vi "Data Access.vi"(8 "error in (no error)":errorcluster, 10 "Data Access Handler":refnum<class "Data Access Handler.lvclass">, 11 "DMM Config Msg in":refnum<class "DMM Config Msg.lvclass">) -> (0 "error out":errorcluster, 3 "DMM Config Msg out":refnum<class "DMM Config Msg.lvclass">)   [LabVIEW 2020, in "DMM Msg.lvlib" / "DMM Config Msg.lvclass"]
doc: "Expose class private data to the front panel while letting the Data Access Handler class act on the data."
uses:
  DMM Config Msg.lvclass
  C:/Current projects/WS/PPL/HDH.Actor Framework.Core.Msg.lvlibp/Flex Msg/Flex Msg.lvclass
  PPL/HDH.Actor Framework.Core.Msg.lvlibp/Flex Msg/Data Access Handlers/Data Access Handler/Data Access Handler.lvclass
  PPL/HDH.Driver.DMM.lvlibp/Controls/Ctl_Function.ctl
  PPL/HDH.Driver.DMM.lvlibp/Controls/Ctl_DigitResolution.ctl
  PPL/HDH.Actor Framework.Core.Publisher.lvlibp/Messages/Response Msg/Response Core/Controls/Ctl_SendFunction.ctl
  DMM Config Msg.lvclass/DMM Config Msg.ctl
  PPL/HDH.Actor Framework.Core.Instrument Handler.lvlibp/Messages/Instrument Msg/Instrument Msg.lvclass
  C:/Current projects/WS/PPL/HDH.Actor Framework.Core.Instrument Handler.lvlibp/Messages/Instrument Msg/Instrument Msg.lvclass
  PPL/HDH.Driver.DMM.lvlibp
  PPL/HDH.Actor Framework.Core.Publisher.lvlibp
panel:
  in  "Message Priority":enum16{"Low", "Normal", "High"}(ring)=enum."Normal"
  in  "Timeout if Waiting":i32=-1
  in  "Send Function":T1=enum."Await Reply"
  in  "Digit Resolution":T2=enum."5½"
  in  "Range":dbl
  in  "Function":T3
  in  "Cancel":bool
  in  "OK":bool
  # "Send details"
  # "Configuration details"
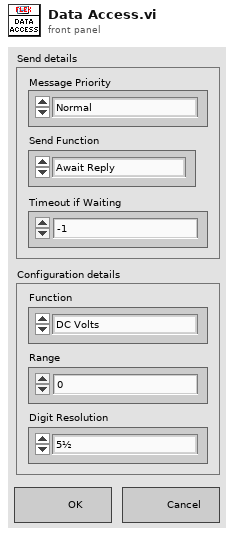
[diagram p1: front panel]
types:
  T1 = typedef "HDH.Actor Framework.Core.Publisher.lvlibp/Ctl_SendFunction.ctl" = enum16{"Send and Forget", "Request Reply", "Await Reply"}
  T2 = typedef "HDH.Driver.DMM.lvlibp/Ctl_DigitResolution.ctl" = enum8{"3½", "4½", "5½", "6½", "7½"}
  T3 = typedef "HDH.Driver.DMM.lvlibp/Ctl_Function.ctl" = enum8{"DC Volts", "AC Volts", "DC Current", "AC Current", "2-wire Resistance", "4-wire Resistance", "Diode", "Frequency", "Period", "AC Volts DC Coupled", "Capacitance", "Inductance", "Temperature"}
  T4 = typedef "HDH.Actor Framework.Core.Actor.lvlibp/Message Enqueuer.lvclass/Message Priority.ctl" = enum16{"Low", "Normal", "High"}
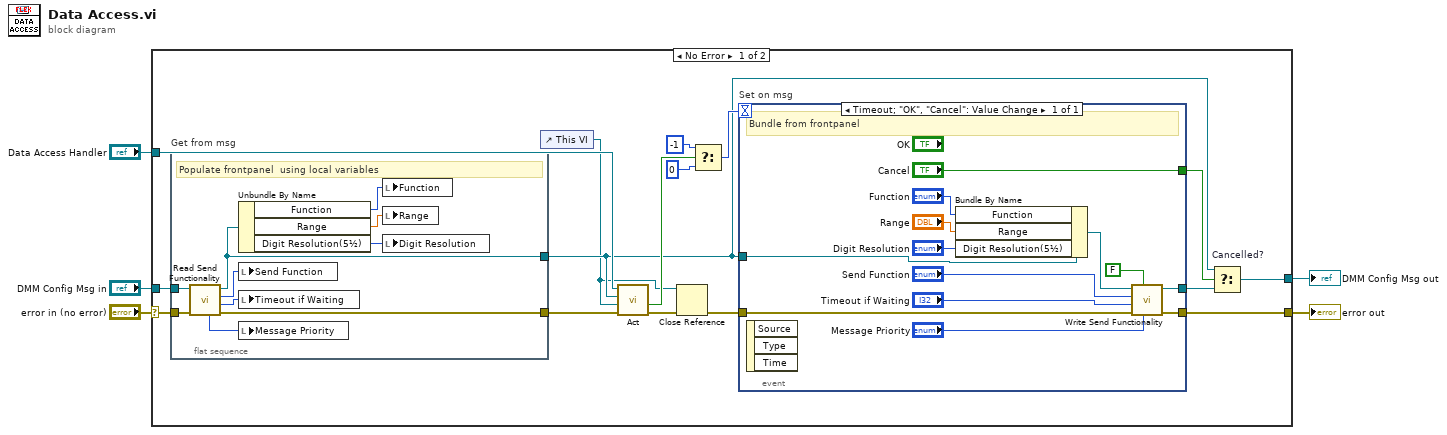
[diagram p0: block diagram]
diagram:
  n1 = case shown="No Error" "error in (no error)" {
    selector: "error in (no error)" -> [w21 w46]
    tunnel: [w14 w46] -> w4
    tunnel: [w9 w45] -> w2
    tunnel: "DMM Config Msg in" -> [w12 w45]
    tunnel: "Data Access Handler" -> [w20 _]
    frame No Error {
      n2 = flat-sequence "Get from msg" {
        tunnel: w21 -> [w43]
        tunnel: [w41] -> w7
        tunnel: w12 -> [w44]
        tunnel: [w42] -> w19
        frame #0 {
          # "Populate frontpanel  using local variables"
          n3 = call "Read Send Functionality.vi"("error in (no error)"=w43, "Instrument Msg in"=w44) -> ("error out"=w42:errorcluster, "Timeout if Waiting"=w36:i32, "Send Function"=w37:T1, "Instrument Msg out"=w41:refnum<class "DMM Config Msg.lvclass">, "Message Priority"=w35:T4)  [unwired: 4 in, 1 out]
          n4 = Unbundle By Name(w41) -> ("Function"=w40:T3, "Range"=w39:dbl, "Digit Resolution(5½)"=w38:T2)
          n5 = local write "Send Function"(w37) -> ()
          n6 = local write "Timeout if Waiting"(w36) -> ()
          n7 = local write "Message Priority"(w35) -> ()
          n8 = local write "Function"(w40) -> ()
          n9 = local write "Range"(w39) -> ()
          n10 = local write "Digit Resolution"(w38) -> ()
        }
      }
      n11 = control-ref of="This VI"() -> (w6:refnum<vi>)
      n12 = call-dynamic "Act.vi"("error in (no error)"=w19, "VI Refnum in"=w6, "Flex Msg type"=w7, "Data Access Handler in"=w20) -> ("error out"=w11:errorcluster, "Await user action?"=w18:bool)  [unwired: 5 in, 1 out]
      n13 = Close Reference(reference=w6, error in (no error)=w11) -> (error out=w13:errorcluster)
      n14 = Select(t=-1, s=w18, f=0 ("t")) -> (s? t:f=w15:i32)
      n15 = event "Set on msg" shown="[0] Timeout;  \"OK\", \"Cancel\": Value Change" {
        selector: _ -> [_]
        dyn-events: _ -> [_]
        timeout: w15 -> [_]
        tunnel: [w26] -> w14
        tunnel: w13 -> [w27]
        tunnel: ["Cancel"] -> w10
        tunnel: [w32] -> w8
        tunnel: w7 -> [w33]
        event Timeout; "OK", "Cancel": Value Change {
          # "Bundle from frontpanel"
          n16 = event-data() -> ()  [unwired: 1 in, 3 out]
          n17 = Bundle By Name(cluster=w33, "Function"="Function", "Range"="Range", "Digit Resolution(5½)"="Digit Resolution") -> (w31:refnum<class "DMM Config Msg.lvclass">)
          n18 = call "Write Send Functionality.vi"("Message Priority(Normal)"="Message Priority", "Publish Data?(T)"=FALSE, "error in (no error)"=w27, "Timeout if Waiting(-1ms)"="Timeout if Waiting", "Send Function(Await Reply)"="Send Function", "Instrument Msg in"=w31) -> ("error out"=w26:errorcluster, "Instrument Msg out"=w32:refnum<class "DMM Config Msg.lvclass">)  [unwired: 4 in]
        }
      }
      n19 = Select "Cancelled?"(t=w7, s=w10, f=w8) -> (s? t:f=w9:refnum<class "DMM Config Msg.lvclass">)
    }
    frame Error {
    }
  }
  "error out" <- w4
  "DMM Config Msg out" <- w2
